vi "Script Name.vi"(8 "error in":errorcluster, 9 "Name":T1, 10 "Name Actor.Terminal Attributes (Init)":T2) -> (0 "error out":errorcluster)   [LabVIEW 2025, in "_Rescript.lvlib" / "Actor.lvlib" / "Actor.lvclass"]
uses:
  Actor.lvclass
  Actor.lvclass/Actor.ctl
  _Rescript.lvlib
  Attributes.ctl
  Terminal Attributes.ctl
  Name.ctl
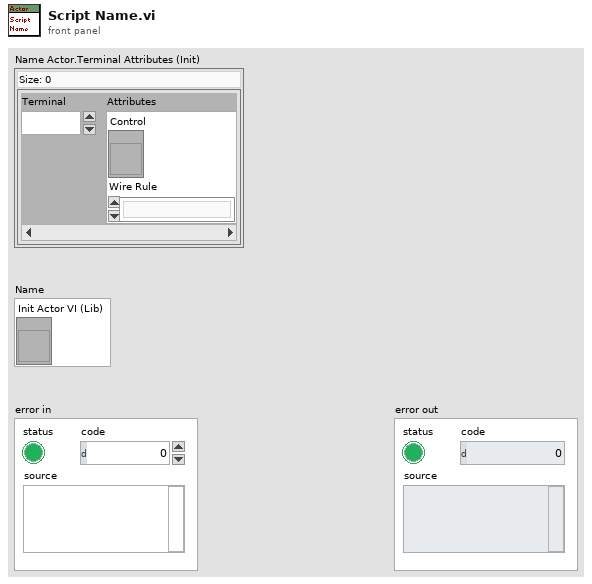
[diagram p1: front panel]
types:
  T1 = typedef "_Rescript.lvlib/Actor.lvlib/Actor.lvclass/Name.ctl" = cluster{"Init Actor VI (Lib)":refnum<vi>}
  T2 = typedef "_Rescript.lvlib/Terminal Attributes.ctl" = map{i32, T3}
  T3 = typedef "_Rescript.lvlib/Attributes.ctl" = cluster{"Control":refnum<vi>, "Wire Rule":enum16{"Invalid Wire Rule", "Required", "Recommended", "Optional", "Dynamic Dispatch"}}
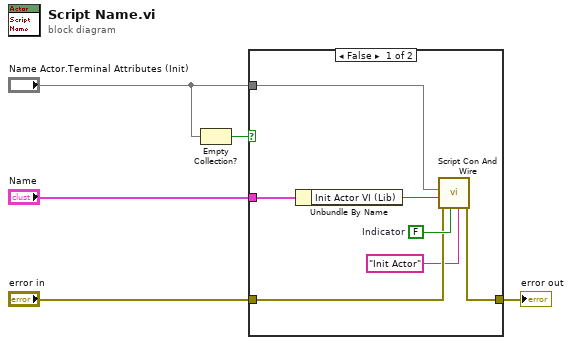
[diagram p0: block diagram]
diagram:
  n1 = Empty Collection?(1:"Name Actor.Terminal Attributes (Init)") -> (0:w5:bool)
  n2 = case shown="False" w5 {
    tunnel: "error in" -> [w9 w13]
    tunnel: "Name" -> [w10 _]
    tunnel: [w7 w13] -> w1
    tunnel: "Name Actor.Terminal Attributes (Init)" -> [w6 _]
    frame False {
      w11 = FALSE  # Indicator
      n3 = Unbundle By Name(w10) -> ("Init Actor VI (Lib)"=w12:refnum<vi>)
      n4 = call "Script Con And Wire.vi"("VI Name"="Init Actor" ("format string"), "Indicator"=w11, "error in"=w9, "VI"=w12, "Terminal Attributes"=w6) -> ("error out"=w7:errorcluster)  [unwired: 6 in]
    }
    frame True {
    }
  }
  "error out" <- w1
